vi "Configure Record Length.vi"(8 "error in (no error)":errorcluster, 9 "Record Length (10000)":i32=10000, 10 "Automatic (T: On)":bool=TRUE, 11 "VISA resource name":refnum<visa-resource-name>) -> (0 "error out":errorcluster, 3 "VISA resource name out":refnum<visa-resource-name>)   [LabVIEW 2020, in "Rohde&Schwarz RTx Oscilloscopes.lvlib"]
doc: "Enables the automatic record length or sets the record length automaticaly.\n\nAttributes:\nRSRTX_ATTR_RECORD_LENGTH_AUTOMATIC\nRSRTX_ATTR_RECORD_LENGTH\n\nRemote-control commands:\nACQuire:POINts:AUTomatic\nACQuire:POINts[:VALue]"
uses:
  Rohde&Schwarz RTx Oscilloscopes.lvlib
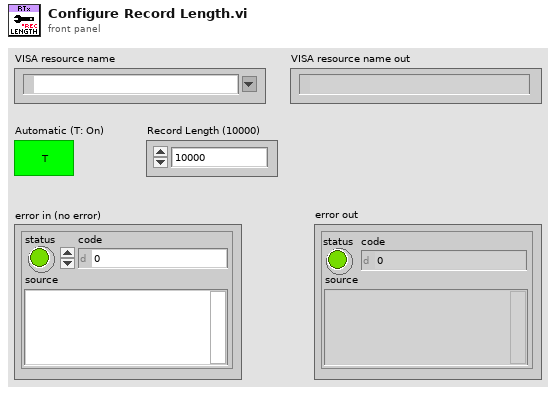
[diagram p1: front panel]
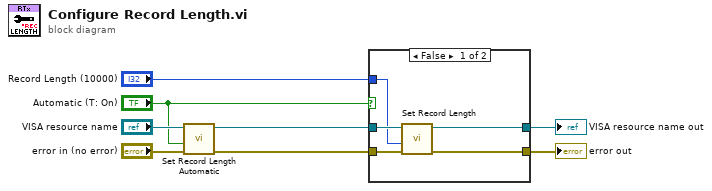
[diagram p0: block diagram]
diagram:
  n1 = call "Set Record Length Automatic"("error in (no error)"="error in (no error)", "Record Length Automatic (OFF)"="Automatic (T: On)", "instrument handle"="VISA resource name") -> ("error out"=w3:errorcluster, "instrument handle out"=w4:refnum<visa-resource-name>)  [unwired: 7 in]
  n2 = case shown="False" "Automatic (T: On)" {
    tunnel: [w13 w14] -> w6
    tunnel: [w12 w15] -> w5
    tunnel: w4 -> [w11 w15]
    tunnel: w3 -> [w10 w14]
    tunnel: "Record Length (10000)" -> [w9 _]
    frame False {
      n3 = call "Set Record Length"("error in (no error)"=w10, "Record Length (0)"=w9, "instrument handle"=w11) -> ("error out"=w13:errorcluster, "instrument handle out"=w12:refnum<visa-resource-name>)  [unwired: 7 in]
    }
    frame True {
    }
  }
  "error out" <- w6
  "VISA resource name out" <- w5
